vi "操作日志.vi"(8 "error in (no error)":errorcluster, 9 "流程参数":string, 10 "日志信息":string, 11 "设备":string="环境动力") -> (0 "error out":errorcluster)   [LabVIEW 2016, in "环境动力监测库.lvlib"]
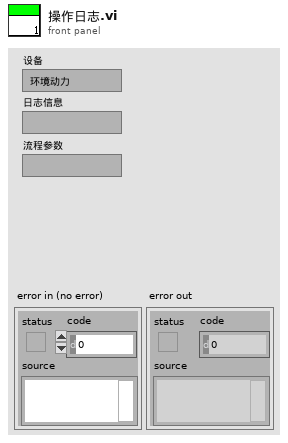
[diagram p1: front panel]
types:
  T1 = typedef "操作日志字段定义.ctl" = cluster{"时间":timestamp, "参数":string, "日志信息":string, "流程参数":string}
  T2 = typedef "数据库类型.ctl" = enum16{"Access", "SQLite"}
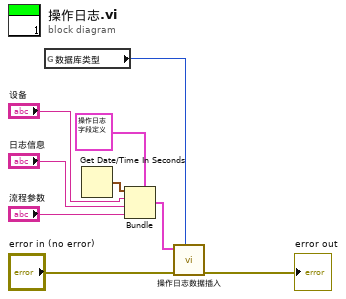
[diagram p0: block diagram]
diagram:
  n1 = global read "断电保存全局变量.vi" "数据库类型"() -> (w3:T2)
  n2 = Get Date/Time In Seconds() -> (seconds since 1Jan1904=w5:timestamp)
  n3 = Bundle(cluster=T1 {"时间"=timestamp(0 s since 1904-01-01), "参数"="水样测试", "日志信息"="N", "流程参数"=""} ("data"), "时间"=w5, "参数"="设备", "日志信息"="日志信息", "流程参数"="流程参数") -> (w4:T1)
  n4 = call "操作日志数据插入.vi"("data"=w4, "错误输入（无错误）"="error in (no error)", "数据库类型"=w3) -> ("错误输出"=→"error out":errorcluster)  [unwired: 7 in]
